vi "DAC Init Results.vi"(8 "error in":errorcluster, 9 "Log Details?":bool, 10 "tdms file":refnum<k34>, 11 "DAC HS Vib in":refnum<class "DAC HS Vib.lvclass">) -> (0 "error out":errorcluster, 2 "tdms file out":refnum<k34>)   [LabVIEW 2019, in "DAC.lvlib" / "DAC HS Vib.lvclass"]
uses:
  DAC HS Vib.lvclass
  C:/Users/krio/Documents/LV_Projects/test-stand/App/DAC/DAC.lvclass
  DAC.lvclass/DAC.ctl
  DAC HS Vib.lvclass/DAC HS Vib.ctl
  DAC.lvclass
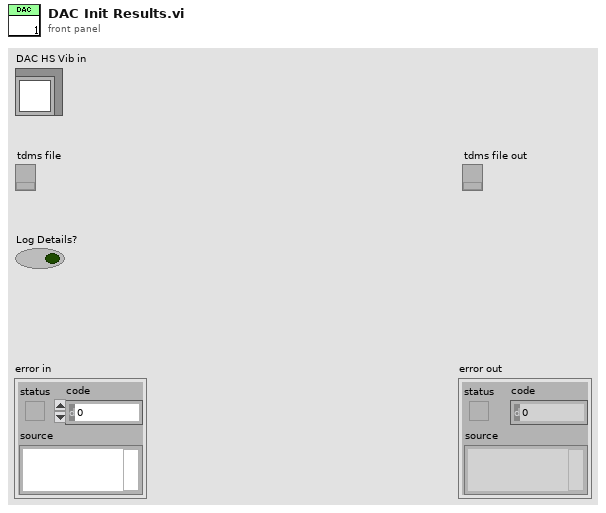
[diagram p1: front panel]
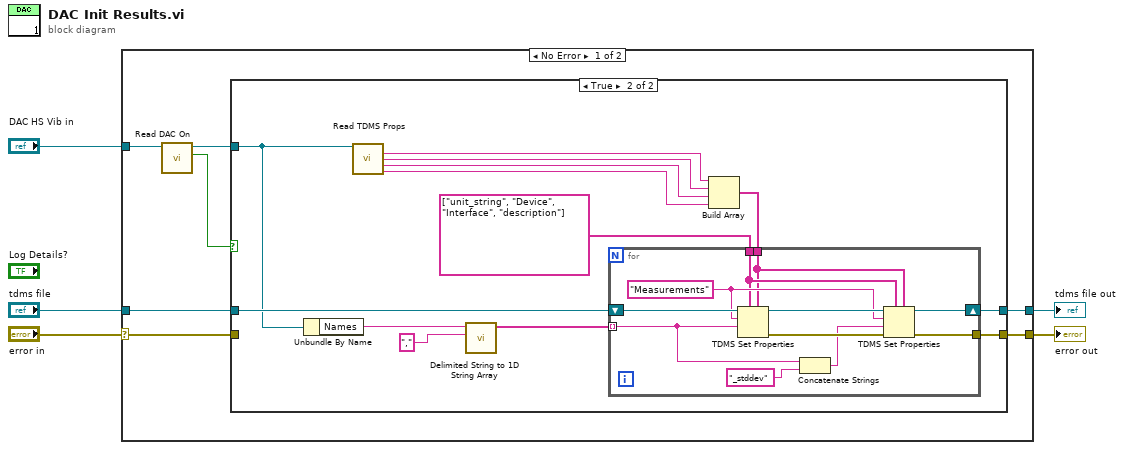
[diagram p0: block diagram]
diagram:
  n1 = case shown="No Error" "error in" {
    selector: "error in" -> [w7 w40]
    tunnel: [w10 w40] -> w2
    tunnel: "DAC HS Vib in" -> [w9 _]
    tunnel: "tdms file" -> [w12 w39]
    tunnel: [w11 w39] -> w1
    frame No Error {
      n2 = call "Read DAC On.vi"("DAC in"=w9) -> ("DAC On"=w6:bool, "DAC out"=w8:refnum<class "DAC HS Vib.lvclass">)  [unwired: 8 in, 1 out]
      n3 = case shown="True" w6 {
        tunnel: w12 -> [w14 w27]
        tunnel: [w14 w26] -> w11
        tunnel: [w13 w25] -> w10
        tunnel: w8 -> [_ w19]
        tunnel: w7 -> [w13 _]
        frame False {
        }
        frame True {
          n4 = Unbundle By Name(w19) -> ("Names"=w22:string)
          n5 = call "Read TDMS Props.vi"("DAC in"=w19) -> ("Result Unit"=w18:string, "DAC Device"=w17:string, "DAC IO"=w16:string, "DAC Description"=w15:string)  [unwired: 10 in, 1 out]
          n6 = call <vilib>:"Delimited String to 1D String Array.vi"("delimiter"=",", "delimited string"=w22) -> ("string array"=w24:string[])  [unwired: 9 in]
          n7 = Build Array(w18, w17, w16, w15) -> (w21:string[])
          n8 = for {
            tunnel: w24 -> [w29] mode=indexing
            tunnel: string[] ["unit_string", "Device", "Interface", "description"] ("property names") -> [w32]
            tunnel: w21 -> [w31]
            tunnel: [w36] -> w25
            shift-right: [w34] -> w26
            shift-left: w27 -> [w38]
            w33 = "Measurements" ("group name in (Untitled)")
            n9 = TDMS Set Properties(5:w31, 7:w32, 9:w29, 10:w33, 11:w38) -> (0:w37:errorcluster, 3:w35:refnum<k34>)  [unwired: 1 in, 2 out]
            n10 = Concatenate Strings(w29, "_stddev" ("string")) -> (w28:string)
            n11 = TDMS Set Properties(5:w31, 7:w32, 8:w37, 9:w28, 10:w33, 11:w35) -> (0:w36:errorcluster, 3:w34:refnum<k34>)  [unwired: 2 out]
          }
        }
      }
    }
    frame Error {
    }
  }
  "error out" <- w2
  "tdms file out" <- w1
